vi "GetMissingDependencies.vi"(8 "error in (no error)":errorcluster, 9 "OutsideVIs in":string[](array[string]), 10 "DestinationDirectory":path, 11 "Project in":refnum<vi>) -> (0 "error out":errorcluster, 3 "OutsideVIs out":string[](array[string]))   [LabVIEW 2021, in "Converter.lvlib"]
uses:
  Converter.lvlib
  e56e842d-5902-469a-bbd5-1077467e5c47.vi
  Converter Reusables/Converter Reusables.lvlib
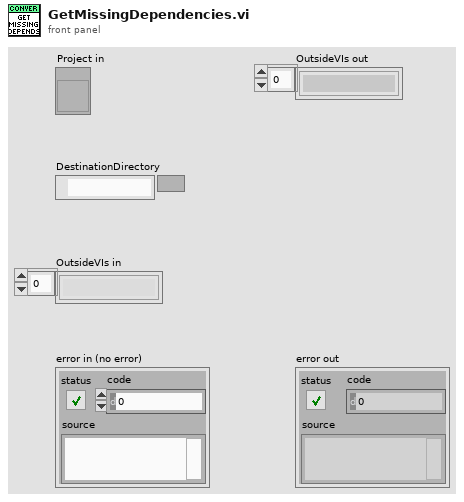
[diagram p1: front panel]
types:
  T1 = typedef "LVMissingDepInfoTypeDef.ctl" = cluster{"Missing Path":path, "Missing Name":string, "Missing Type":string}[]
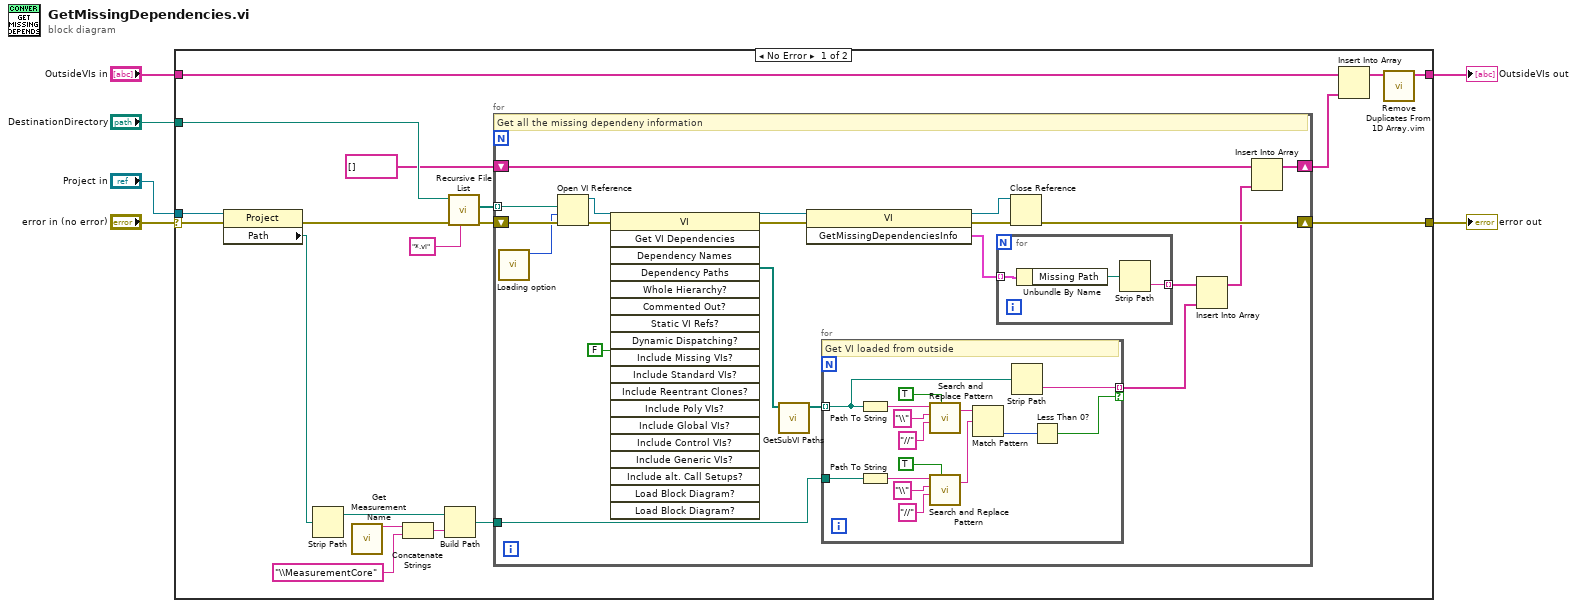
[diagram p0: block diagram]
diagram:
  n1 = case shown="No Error" "error in (no error)" {
    selector: "error in (no error)" -> [w25 w64]
    tunnel: "Project in" -> [w22 _]
    tunnel: [w14 w64] -> w4
    tunnel: "DestinationDirectory" -> [w11 _]
    tunnel: "OutsideVIs in" -> [w9 _]
    tunnel: [w8 _] -> w1
    frame No Error {
      n2 = property class="Project"(reference=w22, error in=w25) -> (error out=w24:errorcluster, "Path"=w23:path)  [unwired: 1 out]
      n3 = Strip Path(path=w23) -> (stripped path=w18:path)  [unwired: 1 out]
      n4 = call "Get Measurement Name.vi"() -> ("Name Out"=w20:string)  [unwired: 14 in, 1 out]
      n5 = Concatenate Strings(w20, "\\MeasurementCore") -> (w17:string)
      n6 = Build Path(base path=w18, name or relative path=w17) -> (appended path=w21:path)
      n7 = call <vilib>:"Recursive File List.vi"("pattern"="*.vi", "error in (no error)"=w24, "Folder Path"=w11) -> ("error out"=w13:errorcluster, "All Files in Dir"=w12:path[])  [unwired: 4 in, 3 out]
      n8 = for {
        tunnel: w12 -> [w45] mode=indexing
        shift-right: [w40] -> w14
        shift-left: w13 -> [w38]
        tunnel: w21 -> [w33]
        shift-right: [w30] -> w16
        shift-left: string[] [] -> [w31]
        # "Get all the missing dependeny information"
        n9 = call "Loading option.vi"() -> ("options"=w26:i32)  [unwired: 11 in]
        n10 = Open VI Reference(vi path=w45, options=w26, error in (no error)=w38) -> (vi reference=w36:refnum<vi>, error out=w44:errorcluster)  [unwired: 3 in]
        n11 = invoke class="VI" method="Get VI Dependencies"(reference=w36, error in=w44, "Include Missing VIs?"=FALSE ("Include Missing Items?")) -> (reference out=w35:refnum<vi>, error out=w37:errorcluster, "Dependency Paths"=w28:path[])  [unwired: 16 in, 16 out]
        n12 = call "GetSubVI Paths.vi"("Dependency Paths"=w28) -> ("ActualDependencies[]"=w27:path[])  [unwired: 9 in, 1 out]
        n13 = invoke class="VI" method="GetMissingDependenciesInfo"(reference=w35, error in=w37) -> (reference out=w39:refnum<vi>, error out=w43:errorcluster, "GetMissingDependenciesInfo"=w42:T1)  [unwired: 1 in]
        n14 = for {
          tunnel: w27 -> [w49] mode=indexing
          tunnel: w33 -> [w50]
          tunnel: [w48] -> w32 mode=indexing if=w46
          # "Get VI loaded from outside"
          n15 = Path To String(path=w49) -> (string=w57:string)
          n16 = Path To String(path=w50) -> (string=w52:string)
          n17 = call <vilib>:"Search and Replace Pattern.vi"("string"=w57, "regular expression (\"\")"="\\" ("search string"), "replace string (\"\")"="//" ("search string"), "replace all? (F)"=TRUE) -> ("result string"=w56:string)  [unwired: 1 in, 1 out]
          n18 = call <vilib>:"Search and Replace Pattern.vi"("string"=w52, "regular expression (\"\")"="\\" ("search string"), "replace string (\"\")"="//" ("search string"), "replace all? (F)"=TRUE) -> ("result string"=w51:string)  [unwired: 1 in, 1 out]
          n19 = Match Pattern(string=w56, regular expression=w51) -> (offset past match=w47:i32)  [unwired: 1 in, 3 out]
          n20 = Strip Path(path=w49) -> (name=w48:string)  [unwired: 1 out]
          n21 = Less Than 0?(x=w47) -> (x < 0?=w46:bool)
        }
        n22 = for {
          tunnel: w42 -> [w63] mode=indexing
          tunnel: [w61] -> w41 mode=indexing
          n23 = Unbundle By Name(w63) -> ("Missing Path"=w62:path)
          n24 = Strip Path(path=w62) -> (name=w61:string)  [unwired: 1 out]
        }
        n25 = Close Reference(reference=w39, error in (no error)=w43) -> (error out=w40:errorcluster)
        n26 = Insert Into Array(array=w41, new element=w32) -> (w29:string[])  [unwired: 1 in]
        n27 = Insert Into Array(array=w31, new element=w29) -> (w30:string[])  [unwired: 1 in]
      }
      n28 = Insert Into Array(array=w9, new element=w16) -> (w15:string[])  [unwired: 1 in]
      n29 = call "Remove Duplicates From 1D Array.vim"("array"=w15) -> ("array with duplicates removed"=w8:string[])  [unwired: 10 in]
    }
    frame Error {
    }
  }
  "OutsideVIs out" <- w1
  "error out" <- w4
